vi "oa_If Param Changed, Set Reset True (N Channels).vi"(0 "scaled signals in [EU]":waveform(dbl)[](array[waveform]), 1 "reset in":bool=TRUE, 5 "speed profile":T1 {"speed [RPM]" format="%.2f"; "time [s]" format="%.2f"}, 7 "pulse/revolution in (1)":i32=1, 9 "max order in (auto)":dbl, 11 "error in (no error)":errorcluster, 12 "analysis method in":u16(ring) items=["fast", "accurate"]) -> (3 "reset out":bool=TRUE, 4 "scaled signals out [EU]":waveform(dbl)[](array[waveform]), 6 "speed profile out":T1 {"speed [RPM]" format="%.2f"; "time [s]" format="%.2f"}, 8 "pulse/revolution out (1)":i32=1, 10 "max order out (auto)":dbl, 14 "analysis method out":u16(ring) items=["fast", "accurate"], 15 "error out":errorcluster)   [LabVIEW 2017, in "SoundVib_Resampling.lvlib"]
uses:
  <vilib>/addons/Sound and Vibration/Order Analysis/Resample Order Tracking/SoundVib_Resampling.lvlib
  <vilib>/addons/Sound and Vibration/Order Analysis/Tach Process/SubVIs/speed profile.ctl
  <vilib>/addons/Sound and Vibration/Order Analysis/Tach Process/SoundVib_TachProcess.lvlib
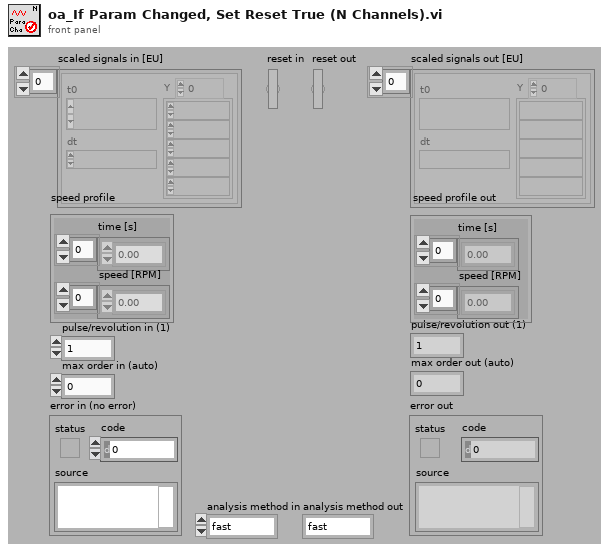
[diagram p1: front panel]
types:
  T1 = typedef "SoundVib_TachProcess.lvlib/speed profile.ctl" = cluster{"time [s]":dbl[], "speed [RPM]":dbl[]}
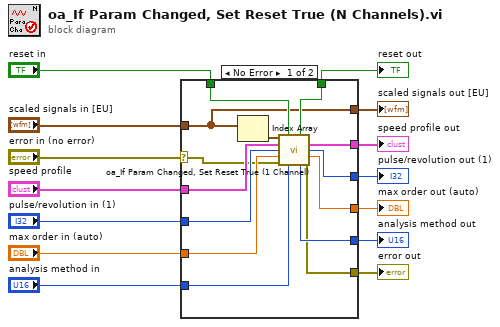
[diagram p0: block diagram]
diagram:
  n1 = case shown="No Error" "error in (no error)" {
    selector: "error in (no error)" -> [w15 w29]
    tunnel: "reset in" -> [w28 w34]
    tunnel: [w27 w34] -> w13
    tunnel: "pulse/revolution in (1)" -> [w25 w31]
    tunnel: "max order in (auto)" -> [w24 w32]
    tunnel: [w23 w31] -> w10
    tunnel: [w22 w32] -> w9
    tunnel: "speed profile" -> [w21 w30]
    tunnel: [w20 w30] -> w7
    tunnel: "analysis method in" -> [w19 w33]
    tunnel: [w18 w33] -> w5
    tunnel: "scaled signals in [EU]" -> [w16 w35]
    tunnel: [w17 w29] -> w4
    tunnel: [w16 w35] -> w3
    frame No Error {
      n2 = Index Array(array=w16) -> (element=w26:waveform(dbl))  [unwired: 1 in]
      n3 = call <vilib>:"oa_If Param Changed, Set Reset True (1 Channel).vi"("scaled signal in [EU]"=w26, "reset in"=w28, "speed profile"=w21, "pulse/revolution in (1)"=w25, "max order in (auto)"=w24, "error in (no error)"=w15, "analysis method in"=w19) -> ("reset out"=w27:bool, "speed profile out"=w20:T1, "pulse/revolution out (1)"=w23:i32, "max order out (auto)"=w22:dbl, "analysis method out"=w18:u16, "error out"=w17:errorcluster)  [unwired: 2 in, 1 out]
    }
    frame Error {
    }
  }
  "reset out" <- w13
  "pulse/revolution out (1)" <- w10
  "analysis method out" <- w5
  "max order out (auto)" <- w9
  "scaled signals out [EU]" <- w3
  "speed profile out" <- w7
  "error out" <- w4
